vi "Clear Specific Error.vi"(8 "error in (no error)":errorcluster, 11 "code":i32) -> (0 "error out":errorcluster, 1 "Cleared?":bool)   [LabVIEW 2011]
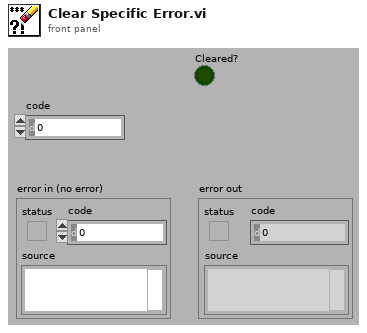
[diagram p1: front panel]
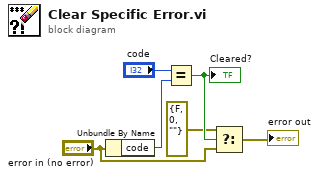
[diagram p0: block diagram]
diagram:
  n1 = Unbundle By Name("error in (no error)") -> ("code"=w5:i32)
  n2 = Equal?(x="code", y=w5) -> (x = y?=w6:bool)
  "Cleared?" <- w6
  n3 = Select(t=errorcluster {"status"=FALSE, "code"=0, "source"=""} ("error in (no error)"), s=w6, f="error in (no error)") -> (s? t:f=→"error out":errorcluster)
